vi "Step 3 - Analyze Quantized Notch (Notch).vi"() -> ()   [LabVIEW 2023]
doc: "Demonstrates how to use the DFD FXP Quantize Coef VI to quantize a notch filter and use the Filter Analysis VIs to analyze the characteristics of the quantized filter.\n\nBefore quantizing the filter coefficients of the notch filter, this example specifies an appropriate filter structure for the target fixed-point notch filter using the DFD Convert Structure VI and scales the filter coefficients using the DFD Scale Filter VI. This example then uses the DFD FXP Quantize Coef VI to quantize the filter coefficients of the notch filter and uses the DFD Plot Freq Response and the DFD Plot Pole-Zero VIs to analyze the quantized notch filter. This example also uses the DFD FXP Coef Report VI to generate a filter coefficients report, which helps you determine if any underflow or overflow occurs during the quantization."
uses:
  <vilib>/addons/Digital Filter Design/_Objects.llb/DFD Pole-Zero Plot.ctl
  <vilib>/addons/Digital Filter Design/Design.llb/DFD IIR Notch Peak Design by Q.vi
  <vilib>/addons/Digital Filter Design/FXPModel.llb/DFD FXP Quantize Coef (Easy).vi
  <vilib>/addons/Digital Filter Design/Analysis.llb/DFD Plot Freq Response (Linear-Spaced).vi
  <vilib>/addons/Digital Filter Design/NI_DigFilterLicensed.lvlib
panel:
  in  "Coefficients b/v Word Length":i16=32
  in  "Coefficients a/k Word Length":i16=32
  in  "Tab Control":enum32{"Magnitude Response", "Pole-Zero"}(tab)
  out "Magnitude Response":cluster{"f0":dbl, "df":dbl, "values":dbl[]}[](graph)
  out "Z-Plane":T1
  out "Coefficients Report":string
  in  "Target Structure":u16(ring)=12 items=["FIR Direct Form"=1, "FIR Direct Form Transposed"=2, "FIR Symmetric"=3, "FIR Antisymmetric"=4, "IIR Direct Form I"=5, "IIR Direct Form I Transposed"=6, "IIR Direct Form II"=7, "IIR Direct Form II Transposed"=8, "IIR Cascaded Second-Order Sections Form I"=9, "IIR Cascaded Second-Order Sections Form I Transposed"=10, "IIR Cascaded Second-Order Sections Form II"=11, "IIR Cascaded Second-Order Sections Form II Transposed"=12, "Lattice Allpass (basic sections)"=13, "Lattice Allpass (one multiplier sections)"=14, "Lattice Allpass (normalized sections)"=15, "Lattice AR (basic sections)"=16, "Lattice AR (one multiplier sections)"=17, "Lattice AR (normalized sections)"=18, "Lattice MA (minimum phase)"=19, "Lattice MA (maximum phase)"=20, "Lattice ARMA (basic sections)"=21, "Lattice ARMA (one multiplier sections)"=22, "Lattice ARMA (normalized sections)"=23]
  # "Select Help>>Show Context Help and move the cursor over the VI icon for more information."
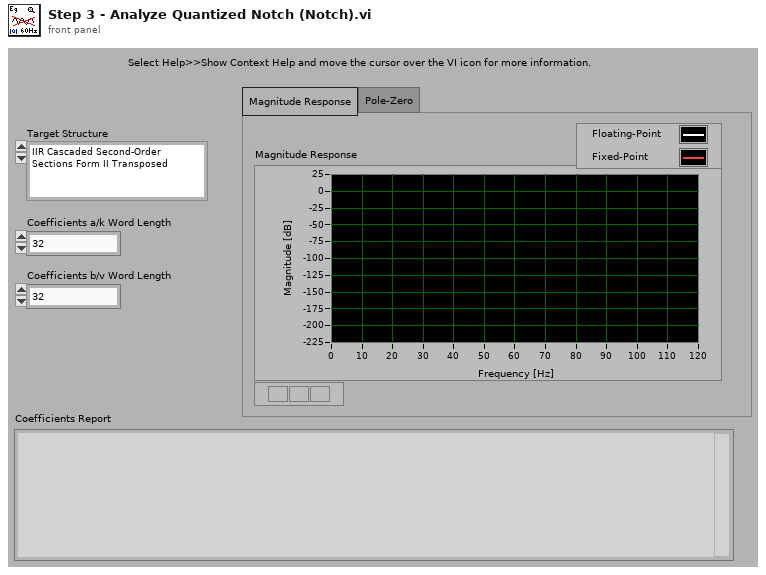
[diagram p1: front panel]
types:
  T1 = typedef "NI_DigFilterLicensed.lvlib/DFD Pole-Zero Plot.ctl" = cluster{dbl[], dbl[]}[]
  T2 = typedef "NI_DigFilterLicensed.lvlib/DFD Filter Obj.ctl" = cluster{"mSRate_Fs":dbl, "mSRate_Version":string, "mSRate_Comments":string, "mSRate_OrgCoef":T3, "mSRate_CurCoef":T3, "mSRate_Quantized?":bool, "mSRate_QCoef":T3, "mSRate_QSettings":T5[], "mSRate_Order":i32, "mSRate_Scaling":cluster{"mSRate_ScaleByPowerOf2?":bool, "mSRate_ScaleType":T7}}
  T3 = typedef "NI_DigFilterLicensed.lvlib/DFD Filter Coef.ctl" = cluster{"type":T4, "gain":dbl, "coef a (k)":dbl[], "coef b (v)":dbl[]}
  T4 = typedef "NI_DigFilterLicensed.lvlib/DFD Filter Structure Type Selector.ctl" = enum16{"Undefined", "FIR Direct Form", "FIR Direct Form Transposed", "FIR Symmetric", "FIR Antisymmetric", "IIR Direct Form I", "IIR Direct Form I Transposed", "IIR Direct Form II", "IIR Direct Form II Transposed", "IIR Cascaded Second Order Sections Form I", "IIR Cascaded Second Order Sections Form I Transposed", "IIR Cascaded Second Order Sections Form II", "IIR Cascaded Second Order Sections Form II Transposed", "Lattice Allpass (basic sections)", "Lattice Allpass (one multiplier sections)", "Lattice Allpass (normalized sections)", "Lattice AR (basic sections)", "Lattice AR (one multiplier sections)", "Lattice AR (normalized sections)", "Lattice MA (minimum phase)", "Lattice MA (maximum phase)", "Lattice ARMA (basic sections)", "Lattice ARMA (one multiplier sections)", "Lattice ARMA (normalized sections)"}
  T5 = typedef "NI_DigFilterLicensed.lvlib/dfd_Internal Quantization Settings.ctl" = cluster{"source":T6, "wl":i16, "iwl":i16, "overflow mode":enum16{"Saturation", "Wrap"}, "rounding mode":enum16{"Nearest", "Truncation"}, "signed?":bool}
  T6 = typedef "NI_DigFilterLicensed.lvlib/dfd_Internal Quantization Srcs.ctl" = u16
  T7 = typedef "NI_DigFilterLicensed.lvlib/DFD Coef Norm Type.ctl" = enum16{"No Norm", "Time Domain 1-Norm", "Time Domain 2-Norm", "Time Domain Inf-Norm"}
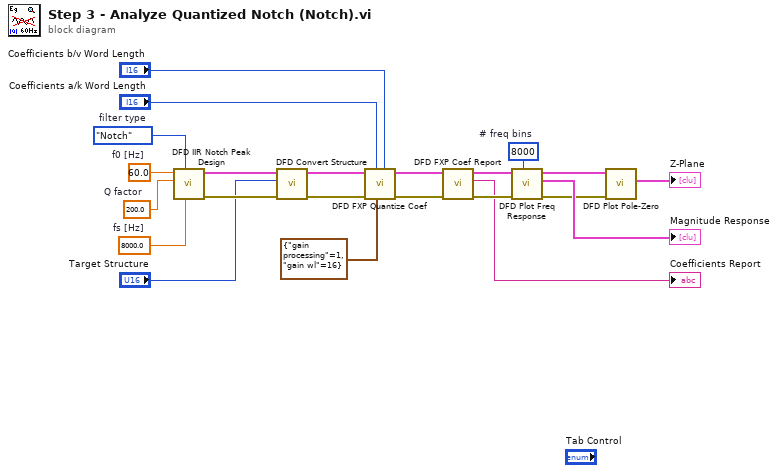
[diagram p0: block diagram]
diagram:
  w2 = 8000  # # freq bins
  w19 = 8000.0  # fs [Hz]
  w20 = 200.0  # Q factor
  w21 = 60.0  # f0 [Hz]
  w22 = enum16{"Notch", "Peak"}."Notch"  # filter type
  n1 = call-poly <vilib>:"DFD IIR Notch Peak Design.vi"("fs [Hz]"=w19, "filter type"=w22, "Q factor"=w20, "f0 [Hz]"=w21) -> ("error out"=w16:errorcluster, "filter out"=w17:T2)  [unwired: 1 in, 5 out]
  n2 = call <vilib>:"DFD Convert Structure.vi"("error in (no error)"=w16, "target structure"="Target Structure", "filter in"=w17) -> ("error out"=w3:errorcluster, "filter out"=w4:T2)  [unwired: 7 out]
  n3 = call-poly <vilib>:"DFD FXP Quantize Coef.vi"("coefficients b/v word length"="Coefficients b/v Word Length", "gain settings"=cluster{"gain processing":u16, "gain wl":i16} {"gain processing"=1, "gain wl"=16}, "coefficients a/k word length"="Coefficients a/k Word Length", "error in (no error)"=w3, "filter in"=w4) -> ("error out"=w11:errorcluster, "filter out"=w12:T2)  [unwired: 5 out]
  n4 = call <vilib>:"DFD FXP Coef Report.vi"("error in (no error)"=w11, "filter in"=w12) -> ("error out"=w9:errorcluster, "coefficients report"=→"Coefficients Report":string, "filter out"=w10:T2)  [unwired: 7 out]
  n5 = call-poly <vilib>:"DFD Plot Freq Response.vi"("# freq bins"=w2, "error in (no error)"=w9, "filter in"=w10) -> ("error out"=w13:errorcluster, "magnitude response"=→"Magnitude Response":cluster{"f0":dbl, "df":dbl, "values":dbl[]}[], "filter out"=w14:T2)  [unwired: 5 in, 1 out]
  n6 = call <vilib>:"DFD Plot Pole-Zero.vi"("error in (no error)"=w13, "filter in"=w14) -> ("Z-Plane"=→"Z-Plane":T1)  [unwired: 1 in, 8 out]
